vi "LinearSystemSim_UpdateY.vi"(8 "MeasurementStdDev":T1, 9 "ClampedU":T1, 10 "X":T1, 11 "Linearsystem":T2) -> (3 "Y":T1)   [LabVIEW 2019, in "Trajectory_Library.lvlib"]
doc: "Creates a new LINEAR SYSTEM data cluster with the specified values. \n\n\nInputs: \n - XXX -- XXX.\n\nOutputs:\n - XXX -- XXX."
uses:
  Trajectory_Library.lvlib
  <vilib>/Analysis/Matrix/Datatypes/RealMatrix.ctl
  LINEAR_SYSTEM.ctl
  <vilib>/Analysis/baseanly.llb/A x B.vi
  <vilib>/Analysis/baseanly.llb/Real A x B.vi
  MatrixHelper_CoerceSize.vi
  MatBuilder_Create.vi
  <vilib>/Analysis/Matrix/Numeric/Add/Add - RM,RM.vi
  <vilib>/Analysis/1siggen.llb/Gaussian White Noise.vi
  <vilib>/Analysis/Matrix/NI_Matrix.lvlib
panel:
  # "<States,States>"
  # "<States,Inputs>"
  # "<Outputs,States>"
  # "<Outputs,Inputs>"
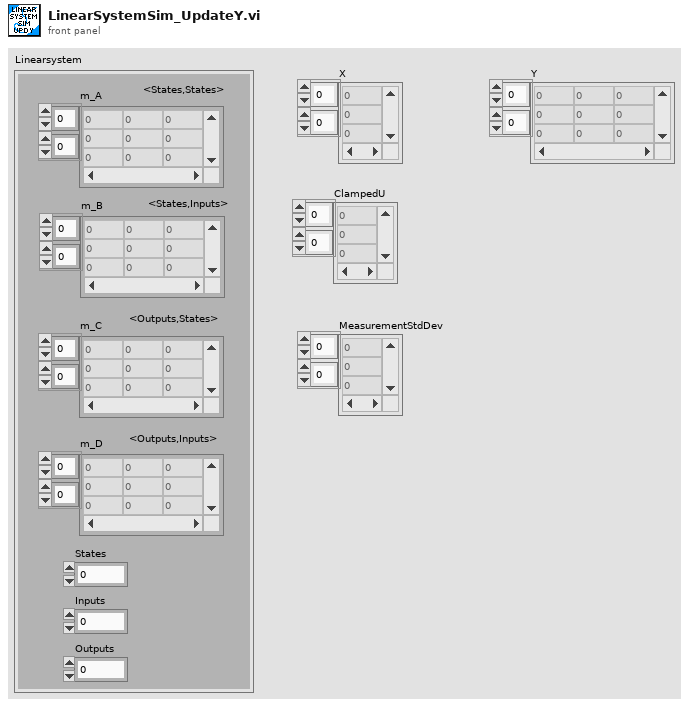
[diagram p1: front panel]
types:
  T1 = typedef "NI_Matrix.lvlib/RealMatrix.ctl" = dbl[][]
  T2 = typedef "Trajectory_Library.lvlib/LINEAR_SYSTEM.ctl" = cluster{"m_A":T1, "m_B":T1, "m_C":T1, "m_D":T1, "States":i32, "Inputs":i32, "Outputs":i32}
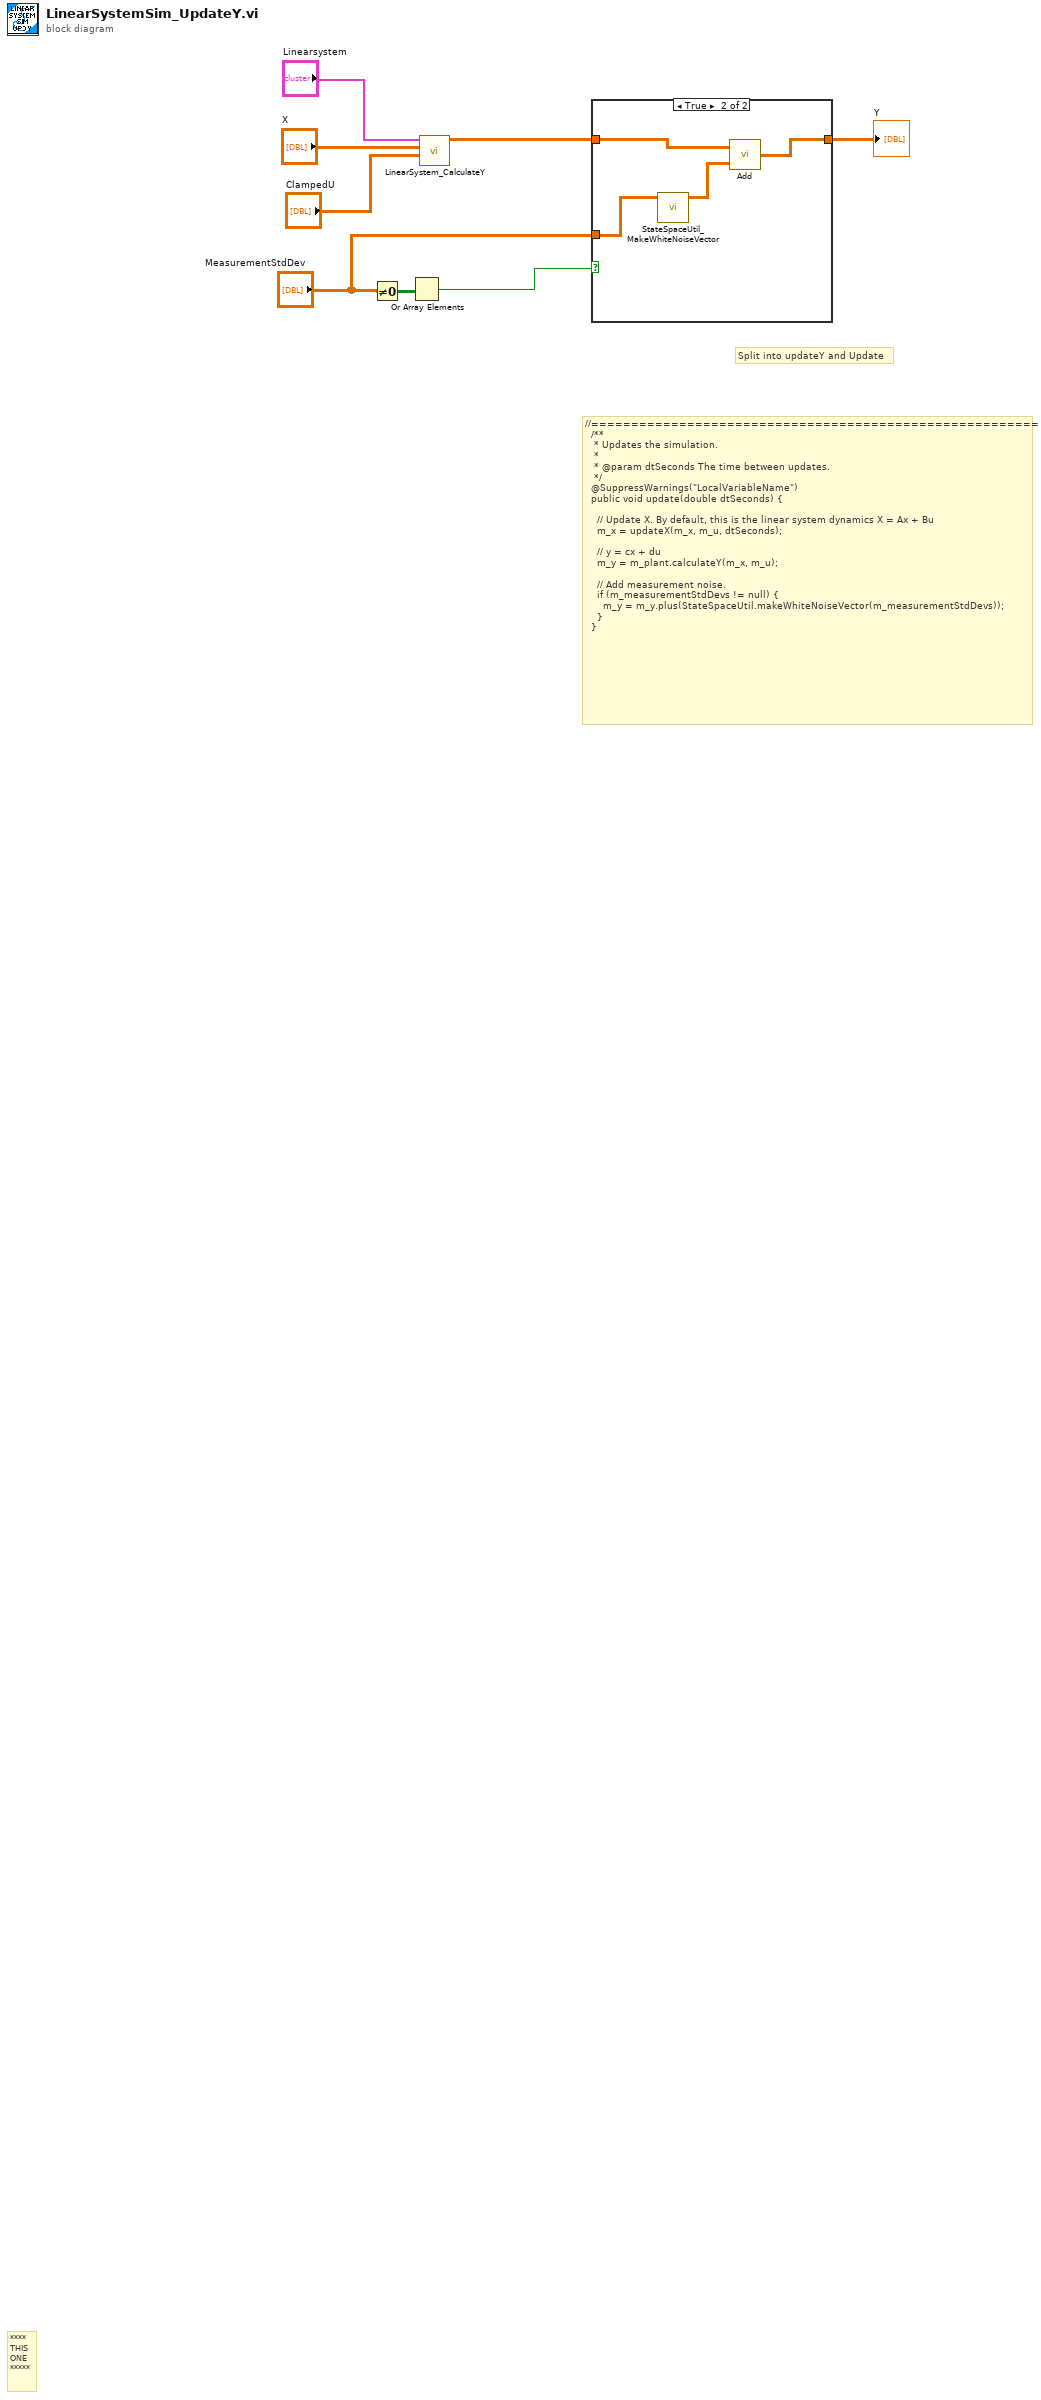
[diagram p0: block diagram]
diagram:
  # "Split into updateY and Update"
  # "//========================================================\n  /**\n   * Updates the simulation.\n   *\n   * @param dtSeconds The time between updates.\n   */\n  @SuppressWarnings(\"LocalVariableName\")\n  public void update(double dtSeconds) {\n\n    // Update X. By default, this is the linear system dynamics X = Ax + Bu\n    m_x = updateX(m_x, m_u, dtSeconds);\n\n    // y = cx + du\n    m_y = m_plant.calculateY(m_x, m_u);\n\n    // Add measurement noise.\n    if (m_measurementStdDevs != null) {\n      m_y = m_y.plus(StateSpaceUtil.makeWhiteNoiseVector(m_measurementStdDevs));\n    }\n  }"
  # "****\nTHIS\nONE\n*****"
  n1 = Not Equal To 0?(x="MeasurementStdDev") -> (x != 0?=w3:bool[][])
  n2 = Or Array Elements(Boolean array=w3) -> (logical OR=w2:bool)
  n3 = call "LinearSystem_CalculateY.vi"("ClampedU"="ClampedU", "X"="X", "Linearsystem"="Linearsystem") -> ("Y"=w8:T1)  [unwired: 7 in, 1 out]
  n4 = case shown="True" w2 {
    tunnel: w8 -> [w9 w12]
    tunnel: [w9 w11] -> w5
    tunnel: "MeasurementStdDev" -> [_ w13]
    frame False {
      # "No Noise"
    }
    frame True {
      n5 = call "StateSpaceUtil_MakeWhiteNoiseVector.vi"("StdDevs"=w13) -> ("WhiteNoise"=w10:T1)  [unwired: 10 in]
      n6 = call-poly <vilib>:"Add.vi"("Real Matrix B"=w10, "Real Matrix A"=w12) -> ("A + B"=w11:T1)
    }
  }
  "Y" <- w5
